vi "add_uint32_roslv.vi"   [LabVIEW 2014]
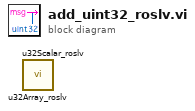
[diagram p0: block diagram]
diagram:
  n1 = call "u32Array_roslv.vi"() -> ()  [unwired: 5 in, 1 out]
  n2 = call "u32Scalar_roslv.vi"() -> ()  [unwired: 5 in, 1 out]
